vi "order1.2018.vi"() -> ()   [LabVIEW 2018]
panel:
  out "Table":string[][](table)
  in  "Boolean":bool
  in  "time":string
  in  "date":string
  in  "scores":dbl
  in  "name":string
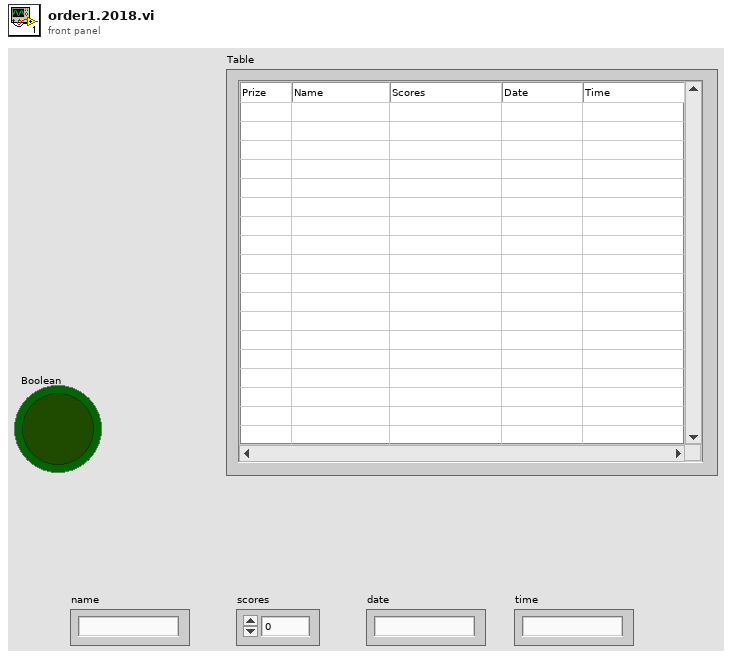
[diagram p1: front panel]
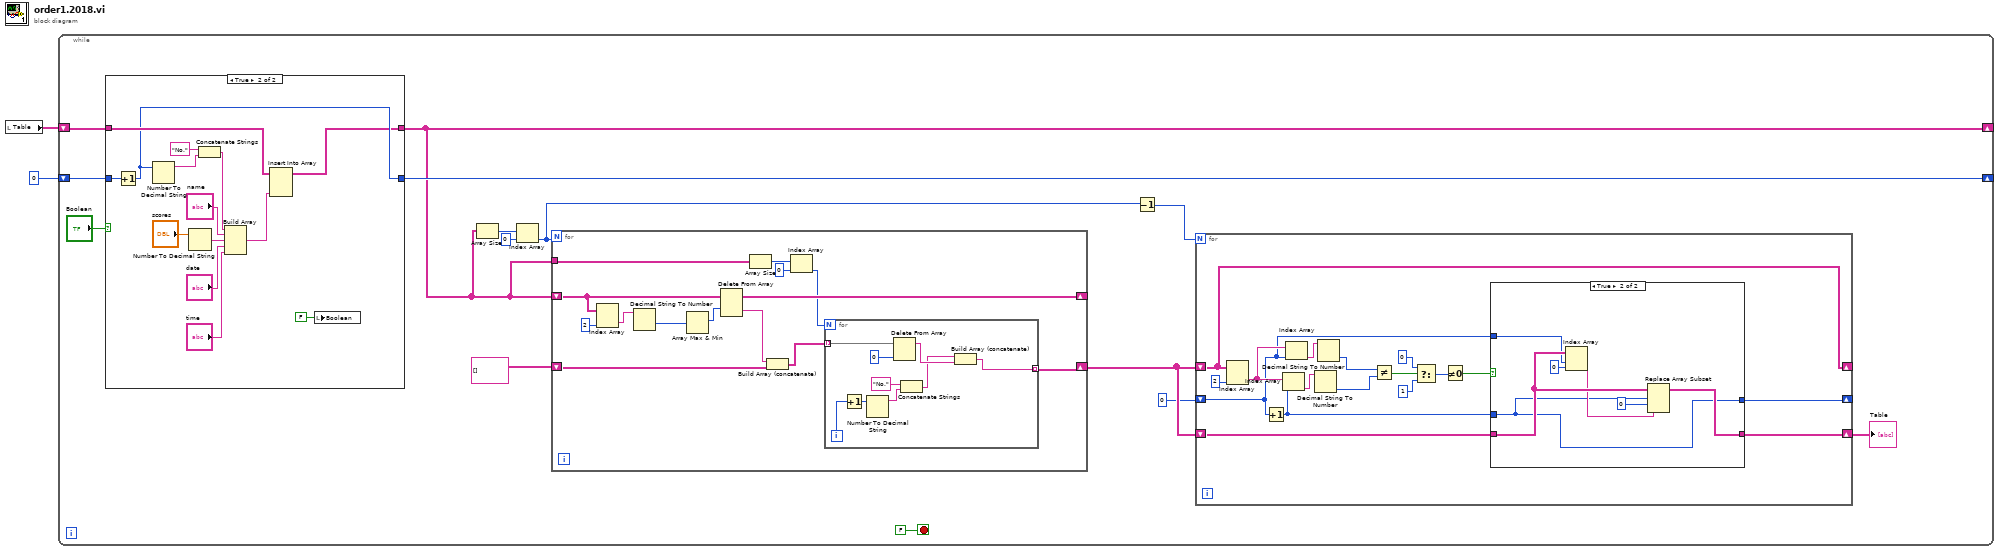
[diagram p0: block diagram]
diagram:
  n1 = local read "Table"() -> (w1:string[][])
  n2 = while {
    shift-right: [w8] -> _
    shift-left: w1 -> [w16]
    shift-right: [w12] -> _
    shift-left: 0 ("index") -> [w13]
    stop <- FALSE stop-if-true
    n3 = case shown="True" "Boolean" {
      tunnel: w16 -> [w67 w75]
      tunnel: [w67 w68] -> w8
      tunnel: w13 -> [w66 w70]
      tunnel: [w66 w69] -> w12
      frame False {
      }
      frame True {
        n4 = Increment(x=w70) -> (x+1=w69:i32)
        n5 = Number To Decimal String(number=w69) -> (decimal integer string=w72:string)  [unwired: 1 in]
        n6 = Number To Decimal String(number="scores") -> (decimal integer string=w79:string)  [unwired: 1 in]
        n7 = Concatenate Strings("No.", w72) -> (w71:string)
        n8 = Build Array(w71, "name", w79, "date", "time") -> (w76:string[])
        n9 = Insert Into Array(array=w75, new element=w76) -> (w68:string[][])  [unwired: 2 in]
        n10 = local write "Boolean"(FALSE ("Boolean")) -> ()
      }
    }
    n11 = Array Size(array=w8) -> (size(s)=w11:i32[])
    n12 = Index Array(array=w11, index=0) -> (element=w7:i32)
    n13 = for {
      N: w7 -> [_]
      shift-right: [w54] -> _
      shift-left: w8 -> [w55]
      shift-right: [w43] -> w6
      shift-left: string[][] [] ("Array") -> [w49]
      tunnel: w8 -> [w46]
      n14 = Index Array(array=w55, index (col)=2 ("disabled index (col)")) -> (element=w52:string[])  [unwired: 1 in]
      n15 = Decimal String To Number(string=w52) -> (number=w51:i32[])  [unwired: 2 in, 1 out]
      n16 = Array Max & Min(array=w51) -> (max index (indices)=w53:i32)  [unwired: 3 out]
      n17 = Delete From Array(array=w55, index (row)=w53) -> (deleted portion=w50:string[], array with subset deleted=w54:string[][])  [unwired: 2 in]
      n18 = Array Size(array=w46) -> (size(s)=w47:i32[])
      n19 = Build Array (concatenate)(w50, w49) -> (w44:string[][])
      n20 = Index Array(array=w47, index=0) -> (element=w45:i32)
      n21 = for {
        N: w45 -> [_]
        tunnel: w44 -> [w63] mode=indexing
        tunnel: [w58] -> w43 mode=indexing
        i -> [w62]
        n22 = Increment(x=w62) -> (x+1=w57:i32)
        n23 = Number To Decimal String(number=w57) -> (decimal integer string=w65:string)  [unwired: 1 in]
        n24 = Delete From Array(array=w63, index=0 ("disabled index (col)")) -> (array with subset deleted=w60:string[])  [unwired: 1 in, 1 out]
        n25 = Concatenate Strings("No.", w65) -> (w59:string)
        n26 = Build Array (concatenate)(w59, w60) -> (w58:string[])
      }
    }
    n27 = Decrement(x=w7) -> (x-1=w4:i32)
    n28 = for {
      N: w4 -> [_]
      shift-right: [w19] -> _
      shift-left: w6 -> [w19]
      shift-right: [w18] -> w3
      shift-left: w6 -> [w30]
      shift-right: [w17] -> _
      shift-left: 0 ("disabled index (col)") -> [w21]
      n29 = Index Array(array=w19, index (col)=2 ("disabled index (col)")) -> (element=w28:string[])  [unwired: 1 in]
      n30 = Increment(x=w21) -> (x+1=w20:i32)
      n31 = Index Array(array=w28, index=w20) -> (element=w32:string)
      n32 = Index Array(array=w28, index=w21) -> (element=w29:string)
      n33 = Decimal String To Number(string=w32) -> (number=w31:i32)  [unwired: 2 in, 1 out]
      n34 = Decimal String To Number(string=w29) -> (number=w27:i32)  [unwired: 2 in, 1 out]
      n35 = Not Equal?(x=w27, y=w31) -> (x != y?=w26:bool)
      n36 = Select(t=0 ("index"), s=w26, f=1 ("index")) -> (s? t:f=w23:i32)
      n37 = Not Equal To 0?(x=w23) -> (x != 0?=w22:bool)
      n38 = case shown="True" w22 {
        tunnel: w30 -> [w35 w41]
        tunnel: w21 -> [_ w37]
        tunnel: w20 -> [w34 w36]
        tunnel: [w35 w38] -> w18
        tunnel: [w34 w36] -> w17
        frame False {
        }
        frame True {
          n39 = Index Array(array=w41, index (row)=w37, index (col)=0 ("disabled index (col)")) -> (element=w39:string)
          n40 = Replace Array Subset(array=w41, new element=w39, index (row)=w36, index (col)=0 ("disabled index (col)")) -> (w38:string[][])
        }
      }
    }
    "Table" <- w3
  }
